vi "TCPServerCycle.vi"   [LabVIEW 2019]
uses:
  02 Mode/TCPServerMode/TCPServerClass.lvclass
types:
  T1 = map{string, refnum<class "TCPServerClass.lvclass">}
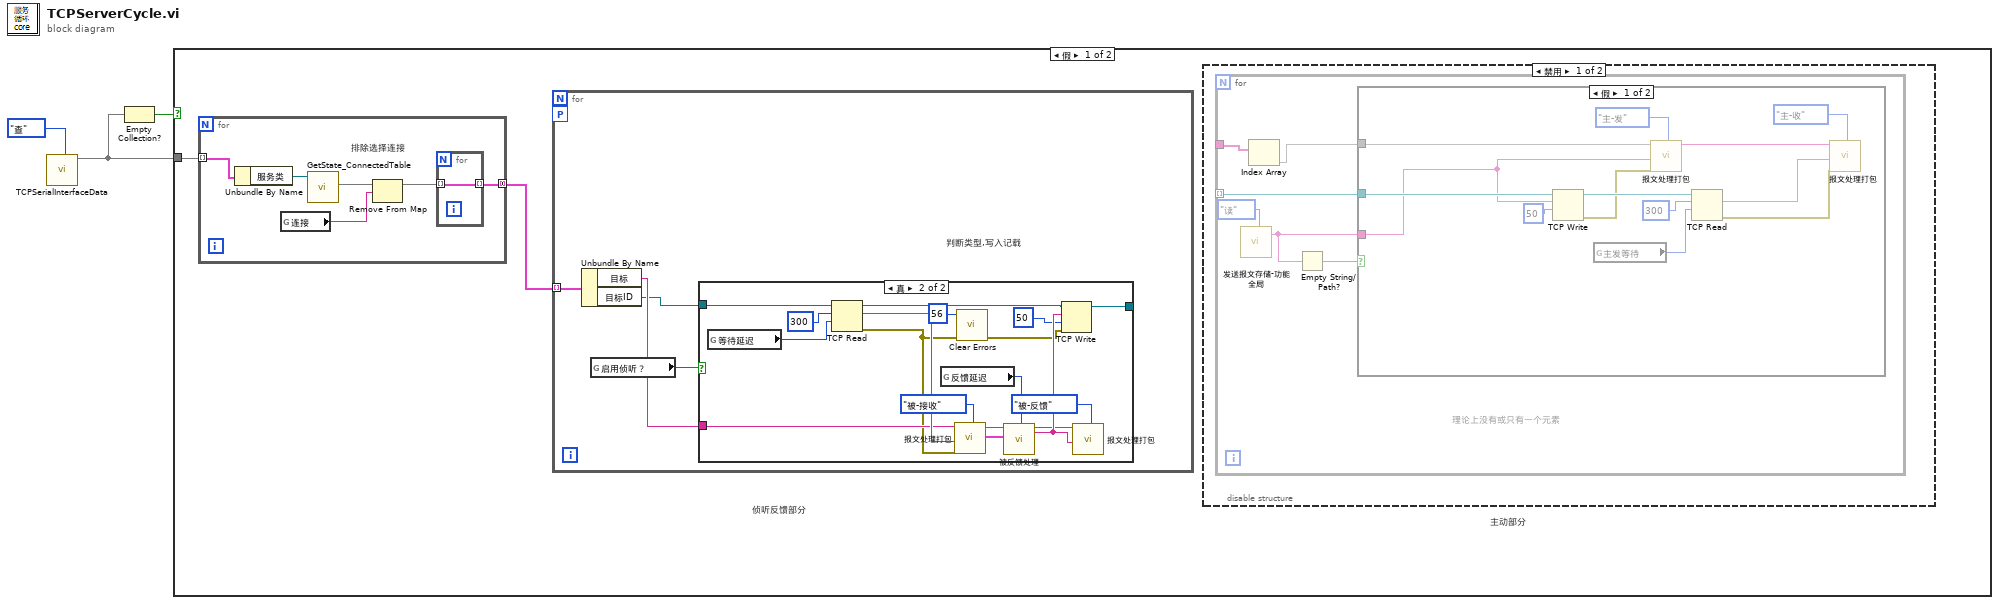
[diagram p0: block diagram]
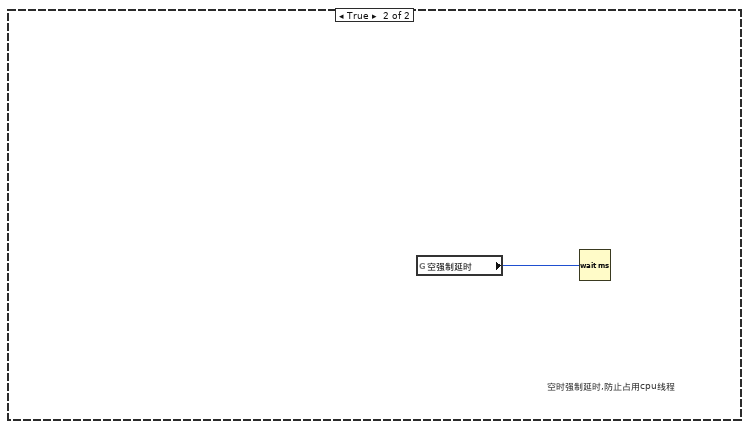
[diagram p5: hidden frame]
diagram:
  n1 = call "TCPSerialInterfaceData.vi"("客服接口枚举"=enum16{"ini", "增", "删", "查", "改", "腾笼换鸟"}."查") -> ("服务表"=w1:T1)  [unwired: 17 in, 1 out]
  n2 = Empty Collection?(1:w1) -> (0:w3:bool)
  n3 = case shown="假" w3 {
    tunnel: w1 -> [w5 _]
    frame False {
      # "主动部分"
      # "侦听反馈部分"
      n4 = for {
        tunnel: w5 -> [w30] mode=indexing
        tunnel: [w28] -> w4 mode=concatenating
        # "排除选择连接"
        n5 = Unbundle By Name(w30) -> ("服务类"=w29:refnum<class "TCPServerClass.lvclass">)
        n6 = global read "全局-配置识别.vi" "连接"() -> (w25:string)
        n7 = call-dynamic "GetState_ConnectedTable.vi"("TCPServerClass输入"=w29) -> ("连接端ID表"=w27:map{string, refnum<k5>})  [unwired: 8 in, 2 out]
        n8 = Remove From Map(10:w25, 11:w27) -> (3:w26:map{string, refnum<k5>})  [unwired: 2 out]
        n9 = for {
          tunnel: [w31] -> w28 mode=indexing
          tunnel: w26 -> [w31] mode=indexing
        }
      }
      n10 = for {
        tunnel: w4 -> [w35] mode=indexing
        workers-P: _ -> [_]
        # "判断类型,写入记载"
        n11 = Unbundle By Name(w35) -> ("目标"=w34:string, "目标ID"=w33:refnum<k5>)
        n12 = global read "全局-被反馈配置.vi" "启用侦听？"() -> (w32:bool)
        n13 = case shown="真" w32 {
          tunnel: [w36 w50] -> _
          tunnel: w34 -> [_ w47]
          tunnel: w33 -> [w36 w46]
          frame False {
          }
          frame True {
            n14 = global read "全局-配置识别.vi" "等待延迟"() -> (w54:u32)
            n15 = TCP Read(connection ID=w46, bytes to read=300 ("读取的字节"), 9:w54) -> (connection ID out=w51:refnum<k5>, data out=w49:string, error out=w39:errorcluster)  [unwired: 2 in]
            n16 = global read "全局-配置识别.vi" "反馈延迟"() -> (w40:u32)
            n17 = call "报文处理打包.vi"("识别名称"=w47, "报文"=w49, "Error In"=w39, "类型"=enum16{"被-接收", "被-反馈", "主-发", "主-收"}."被-接收") -> ("识别名称输出"=w44:string, "被收校验信息"=w43:cluster{"可用？":bool, "功能码":u8, "无crc报文":u8[]})  [unwired: 14 in]
            n18 = call <vilib>:"Clear Errors.vi"("error in (no error)"=w39, "specific error code to clear (0: all)"=56) -> ("error out"=w37:errorcluster)  [unwired: 4 in, 1 out]
            n19 = call "被反馈处理.vi"("识别名称"=w44, "校验信息"=w43, "等待时间（毫秒）"=w40) -> ("识别名称输出"=w42:string, "反馈"=w52:string)  [unwired: 15 in]
            n20 = TCP Write(connection ID=w51, data in=w52, error in (no error)=w37, 9:50 ("超时毫秒(25000)")) -> (connection ID out=w50:refnum<k5>)  [unwired: 2 out]
            n21 = call "报文处理打包.vi"("识别名称"=w42, "报文"=w52, "类型"=enum16{"被-接收", "被-反馈", "主-发", "主-收"}."被-反馈") -> ()  [unwired: 15 in, 2 out]
          }
        }
      }
      n22 = disable-structure shown="禁用" {
        frame Disabled {
          n23 = for {
            tunnel: _ -> [w11] mode=indexing
            tunnel: _ -> [w7]
            # "理论上没有或只有一个元素"
            n24 = call "发送报文存储-功能全局.vi"("枚举"=enum16{"ini", "读", "写"}."读") -> ("报文输出"=w8:string)  [unwired: 18 in]
            n25 = Index Array(array=w7) -> (element=w6)  [unwired: 1 in]
            n26 = Empty String/Path?(string/path=w8) -> (empty?=w9:bool)
            n27 = case shown="假" w9 {
              tunnel: w11 -> [w24 _]
              tunnel: w8 -> [w19 _]
              tunnel: w6 -> [w20 _]
              frame False {
                n28 = TCP Write(connection ID=w24, data in=w19, 9:50 ("超时毫秒(25000)")) -> (connection ID out=w17:refnum<k5>, error out=w16:errorcluster)  [unwired: 1 in, 1 out]
                n29 = global read "全局-配置识别.vi" "主发等待"() -> (w15:u32)
                n30 = call "报文处理打包.vi"("识别名称"=w20, "报文"=w19, "Error In"=w16, "类型"=enum16{"被-接收", "被-反馈", "主-发", "主-收"}."主-发") -> ("识别名称输出"=w21:string)  [unwired: 14 in, 1 out]
                n31 = TCP Read(connection ID=w17, bytes to read=300 ("读取的字节"), 9:w15) -> (data out=w12:string, error out=w13:errorcluster)  [unwired: 2 in, 1 out]
                n32 = call "报文处理打包.vi"("识别名称"=w21, "报文"=w12, "Error In"=w13, "类型"=enum16{"被-接收", "被-反馈", "主-发", "主-收"}."主-收") -> ()  [unwired: 14 in, 2 out]
              }
              frame True {
              }
            }
          }
        }
        frame Enabled {
        }
      }
    }
    frame True {
      # "空时强制延时,防止占用cpu线程"
      n33 = global read "全局-配置识别.vi" "空强制延时"() -> (w55:u32)
      n34 = Wait (ms)(milliseconds to wait=w55) -> ()  [unwired: 1 out]
    }
  }
